vi "While Loops.vi"() -> ()   [LabVIEW 2019]
panel:
  out "Numeric":i32
  in  "stop":bool
  out "number (0 to 1)":dbl
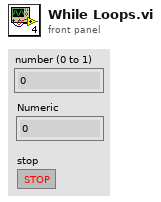
[diagram p1: front panel]
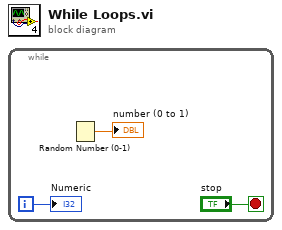
[diagram p0: block diagram]
diagram:
  n1 = while {
    i -> [w1]
    stop <- "stop" stop-if-true
    n2 = Random Number (0-1)() -> (number: 0 to 1=→"number (0 to 1)":dbl)
    "Numeric" <- w1
  }
